vi "ArrayFormer.vi"(2 "New Data":dbl, 3 "stop":bool, 4 "Existing":dbl[](array[numeric])) -> (0 "Current":dbl[](array[numeric]), 1 "Average":dbl)   [LabVIEW 2012]
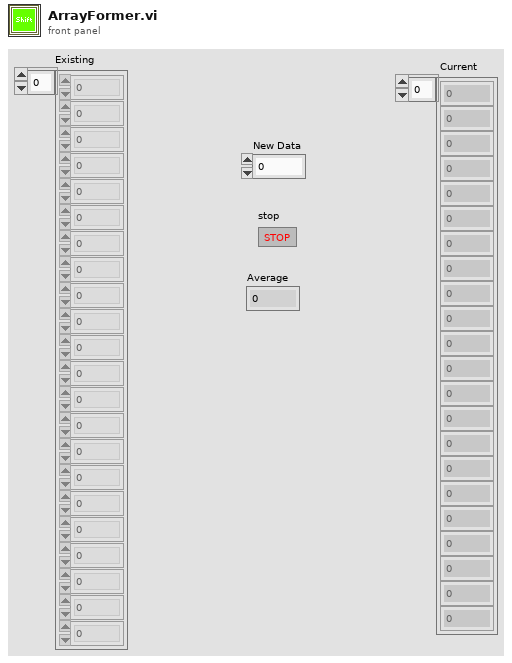
[diagram p1: front panel]
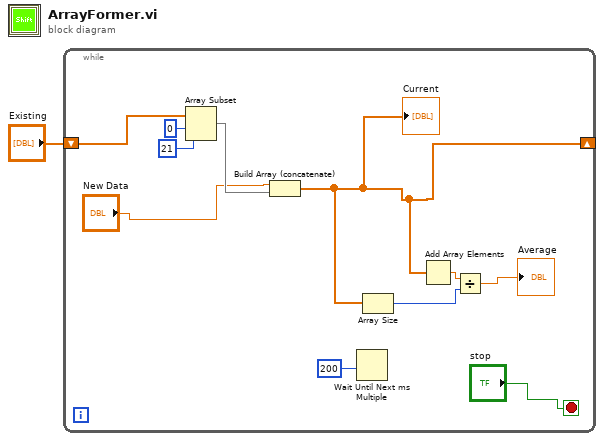
[diagram p0: block diagram]
diagram:
  n1 = while {
    shift-right: [w3] -> _
    shift-left: "Existing" -> [w12]
    stop <- "stop" stop-if-true
    n2 = Array Subset(array=w12, index=0, length=21) -> (w9:dbl[])
    n3 = Build Array (concatenate)("New Data", w9) -> (w3:dbl[])
    "Current" <- w3
    n4 = Wait Until Next ms Multiple(millisecond multiple=200) -> ()  [unwired: 1 out]
    n5 = Array Size(array=w3) -> (size(s)=w2:i32)
    n6 = Add Array Elements(numeric array=w3) -> (sum=w5:dbl)
    n7 = Divide(x=w5, y=w2) -> (x/y=→"Average":dbl)
  }
